vi "SmallestAngle.vi"(10 "Angle B":dbl, 11 "Angle A":dbl) -> (3 "Smallest B to A":dbl)   [LabVIEW 2016]
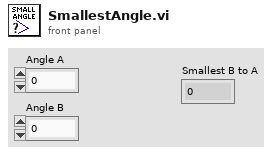
[diagram p1: front panel]
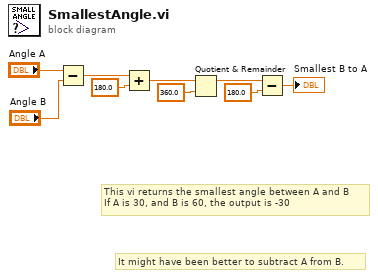
[diagram p0: block diagram]
diagram:
  # "It might have been better to subtract A from B."
  # "This vi returns the smallest angle between A and B\nIf A is 30, and B is 60, the output is -30"
  n1 = Subtract(x="Angle A", y="Angle B") -> (x-y=w7:dbl)
  n2 = Add(x=w7, y=180.0) -> (x+y=w5:dbl)
  n3 = Quotient & Remainder(x=w5, y=360.0) -> (x-y*floor(x/y)=w3:dbl)  [unwired: 1 out]
  n4 = Subtract(x=w3, y=180.0) -> (x-y=→"Smallest B to A":dbl)
